vi "Ball Index (SubVI).vi"(4 "cur pos Y":sgl, 5 "cur pos X":sgl, 6 "Circles Calibrated (Shape Detection 1)":T1(array[cluster]) {"Position"."Y" format="%.2f"; "Position"."X" format="%.2f"}, 7 "Ball index":i32, 8 "reference in":refnum<vi>, 9 "Digital in":refnum<vi>) -> ()   [LabVIEW 2017]
panel:
  in  "Range":sgl=20.0
  in  "last pos Y":sgl
  in  "last pos X":sgl
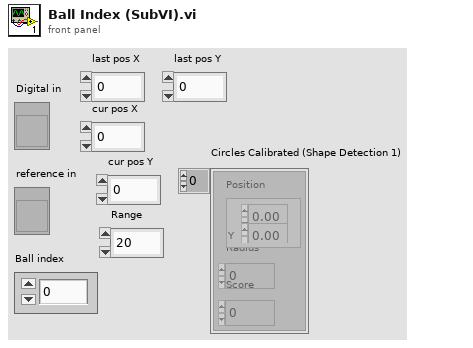
[diagram p1: front panel]
types:
  T1 = cluster{"Position":cluster{"X":sgl, "Y":sgl}, "Radius":dbl, "Score":dbl}[]
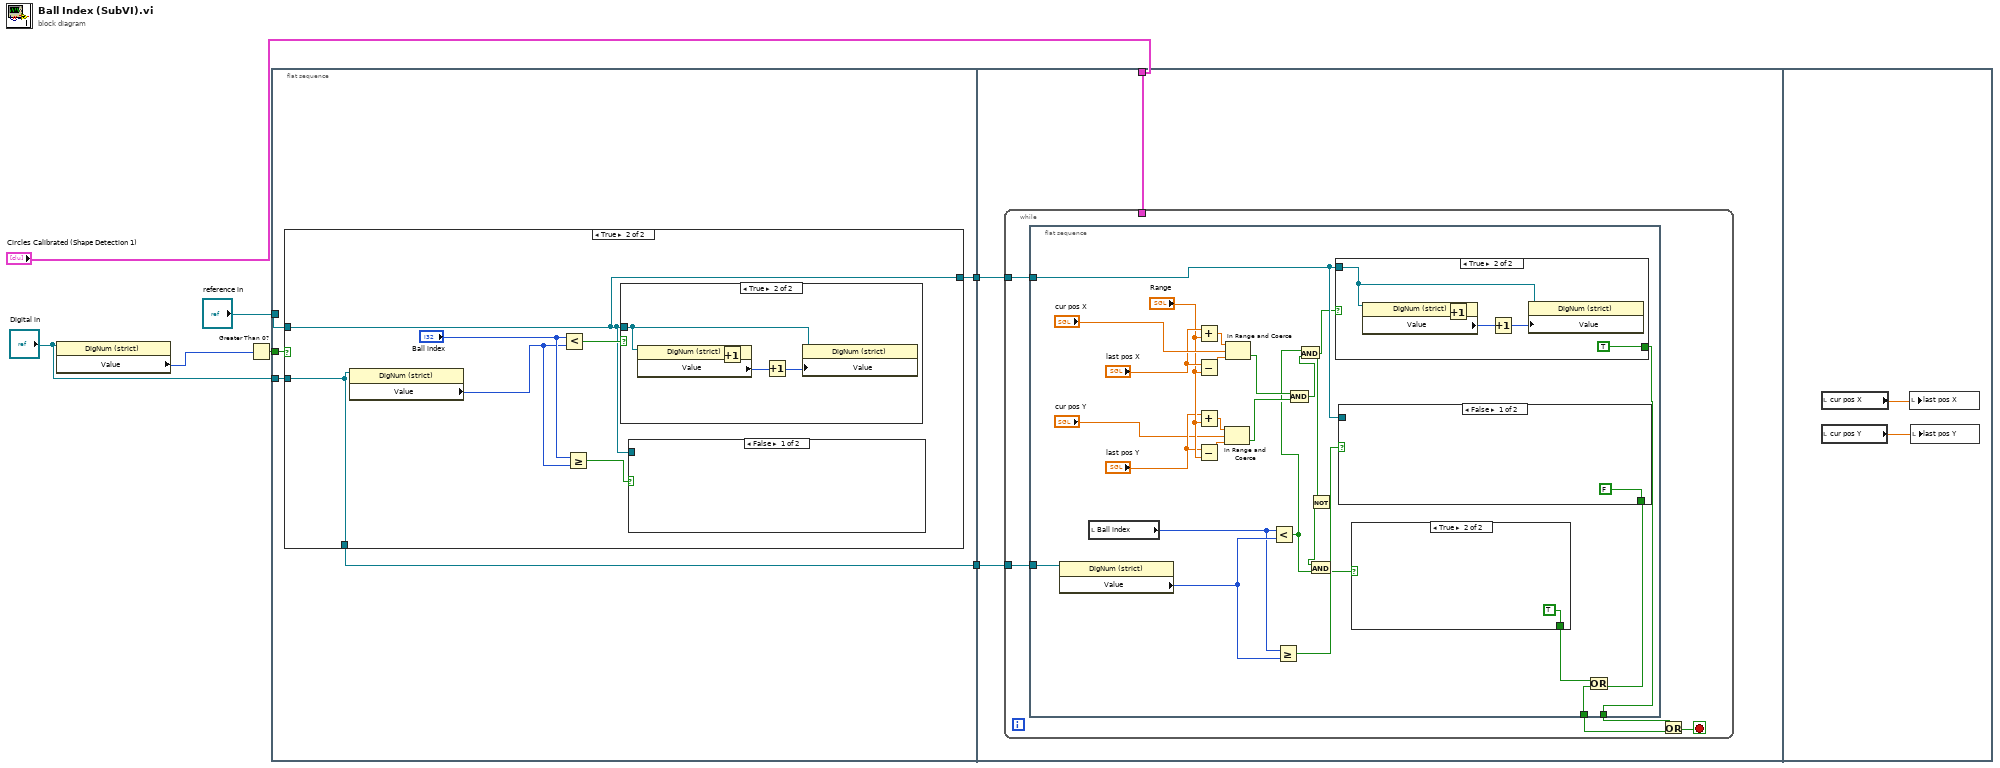
[diagram p0: block diagram]
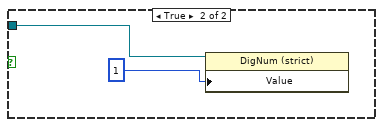
[diagram p3: hidden frame]
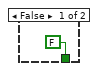
[diagram p5: hidden frame]
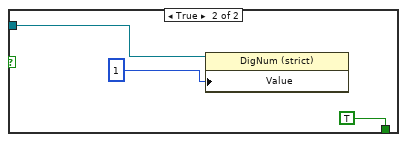
[diagram p6: hidden frame]
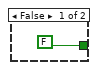
[diagram p7: hidden frame]
diagram:
  n1 = property class="DigNum (strict)"(reference="Digital in") -> ("Value"=w6:i32)  [unwired: 1 in, 2 out]
  n2 = Greater Than 0?(x=w6) -> (x > 0?=w7:bool)
  n3 = flat-sequence {
    tunnel: w7 -> [w12]
    tunnel: "reference in" -> [w11]
    tunnel: "Digital in" -> [w10]
    tunnel: [w9] -> w3
    tunnel: [w8] -> w1
    tunnel: w3 -> [w28]
    tunnel: "Circles Calibrated (Shape Detection 1)" -> [w27]
    tunnel: w1 -> [w26]
    frame #0 {
      n4 = case shown="True" w12 {
        tunnel: w11 -> [w14 w16]
        tunnel: w10 -> [w13 w15]
        tunnel: [w14 w16] -> w9
        tunnel: [w13 w15] -> w8
        frame False {
        }
        frame True {
          n5 = property class="DigNum (strict)"(reference=w15) -> ("Value"=w18:i32)  [unwired: 1 in, 2 out]
          n6 = Less?(x="Ball index", y=w18) -> (x < y?=w20:bool)
          n7 = Greater Or Equal?(x="Ball index", y=w18) -> (x >= y?=w17:bool)
          n8 = case shown="True" w20 {
            tunnel: w16 -> [_ w25]
            frame False {
            }
            frame True {
              n9 = property class="DigNum (strict)"(reference=w25) -> ("Value"=w24:i32)  [unwired: 1 in, 2 out]
              n10 = Increment(x=w24) -> ()  [unwired: 1 out]
              n11 = Increment(x=w24) -> (x+1=w23:i32)
              n12 = property class="DigNum (strict)"(reference=w25, "Value"=w23) -> ()  [unwired: 1 in, 2 out]
            }
          }
          n13 = case shown="False" w17 {
            tunnel: w16 -> [_ w22]
            frame False {
            }
            frame True {
              n14 = property class="DigNum (strict)"(reference=w22, "Value"=1 ("Ball index")) -> ()  [unwired: 1 in, 2 out]
            }
          }
        }
      }
    }
    frame #1 {
      n15 = while {
        tunnel: w28 -> [w33]
        tunnel: w27 -> [_]
        tunnel: w26 -> [w31]
        stop <- w30 stop-if-true
        n16 = flat-sequence {
          tunnel: [w38] -> w32
          tunnel: [w41] -> w29
          tunnel: w33 -> [w46]
          tunnel: w31 -> [w42]
          frame #0 {
            n17 = property class="DigNum (strict)"(reference=w42) -> ("Value"=w45:i32)  [unwired: 1 in, 2 out]
            n18 = local read "Ball index"() -> (w44:i32)
            n19 = Add(x="last pos X", y="Range") -> (x+y=w57:sgl)
            n20 = Subtract(x="last pos X", y="Range") -> (x-y=w58:sgl)
            n21 = Add(x="last pos Y", y="Range") -> (x+y=w53:sgl)
            n22 = Subtract(x="last pos Y", y="Range") -> (x-y=w54:sgl)
            n23 = In Range and Coerce(upper limit=w53, x="cur pos Y", lower limit=w54) -> (In Range?=w48:bool)  [unwired: 1 out]
            n24 = In Range and Coerce(upper limit=w57, x="cur pos X", lower limit=w58) -> (In Range?=w49:bool)  [unwired: 1 out]
            n25 = Less?(x=w44, y=w45) -> (x < y?=w39:bool)
            n26 = Greater Or Equal?(x=w44, y=w45) -> (x >= y?=w43:bool)
            n27 = And(x=w49, y=w48) -> (x .and. y?=w47:bool)
            n28 = And(x=w39, y=w47) -> (x .and. y?=w35:bool)
            n29 = Not(x=w35) -> (.not. x?=w34:bool)
            n30 = And(x=w34, y=w39) -> (x .and. y?=w36:bool)
            n31 = case shown="True" w35 {
              tunnel: w46 -> [_ w67]
              tunnel: [FALSE TRUE] -> w41
              frame False {
              }
              frame True {
                n32 = property class="DigNum (strict)"(reference=w67) -> ("Value"=w69:i32)  [unwired: 1 in, 2 out]
                n33 = Increment(x=w69) -> ()  [unwired: 1 out]
                n34 = Increment(x=w69) -> (x+1=w68:i32)
                n35 = property class="DigNum (strict)"(reference=w67, "Value"=w68) -> ()  [unwired: 1 in, 2 out]
              }
            }
            n36 = case shown="False" w43 {
              tunnel: w46 -> [_ w64]
              tunnel: [FALSE TRUE] -> w40
              frame False {
              }
              frame True {
                n37 = property class="DigNum (strict)"(reference=w64, "Value"=1 ("Ball index")) -> ()  [unwired: 1 in, 2 out]
              }
            }
            n38 = case shown="True" w36 {
              tunnel: [FALSE TRUE] -> w37
              frame False {
              }
              frame True {
              }
            }
            n39 = Or(x=w37, y=w40) -> (x .or. y?=w38:bool)
          }
        }
        n40 = Or(x=w29, y=w32) -> (x .or. y?=w30:bool)
      }
    }
    frame #2 {
      n41 = local read "cur pos X"() -> (w71:sgl)
      n42 = local read "cur pos Y"() -> (w70:sgl)
      n43 = local write "last pos X"(w71) -> ()
      n44 = local write "last pos Y"(w70) -> ()
    }
  }
